vi "MB Serial Example Slave.vi"() -> ()   [LabVIEW 2019, in "NI_modbus_upd.lvlib"]
uses:
  NI_modbus_upd.lvlib
  MB Globals.vi
panel:
  in  "Stop":bool
  out "Holding Registers":u16[](array[numeric]) caption="Holding Registers (Master can write in these registers)"
  out "Coils":bool[](array[boolean]) caption="Coils (Master can write coils)"
  in  "Discrete Inputs":bool[](array[boolean]) caption="Discrete Inputs (Master can only read them)"
  in  "Input Registers":u16[](array[numeric]) caption="Input Registers (Master can only read them)"
  in  "VISA resource name":refnum<visa-resource-name>
  # "MB Serial Example Slave.vi\n\nInstructions\n1. Connect your 2 COMs ports using a cross-over cable\n2. Select a COM port in VISA resouce name\n3. Run the VI\n4. Open and run MB Example Master.vi\n5. Modify the discrete inputs or input registers on the slave -> they're updated on the master.\n6. Modify the coils and registers on the master -> they're updated on the slave."
  # "Slave Registers"
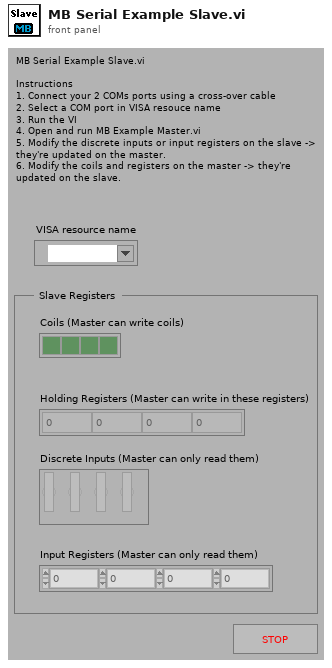
[diagram p1: front panel]
types:
  T1 = enum16{"Discrete Inputs", "Coils", "Input Registers", "Holding Registers"}
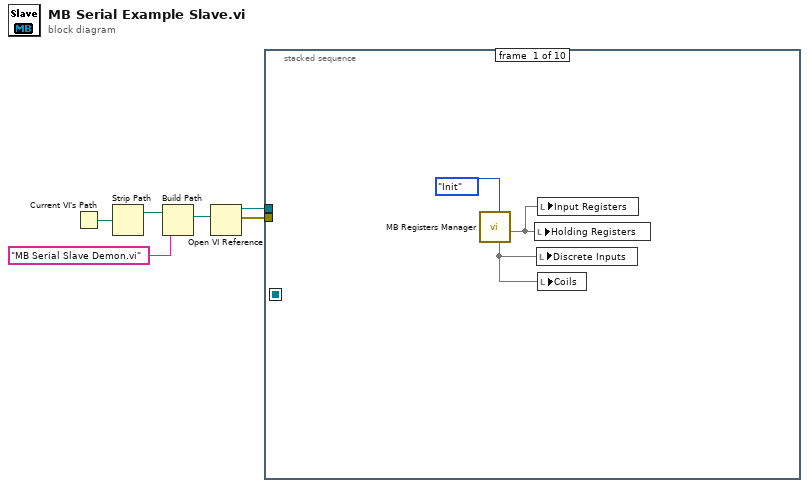
[diagram p0: block diagram]
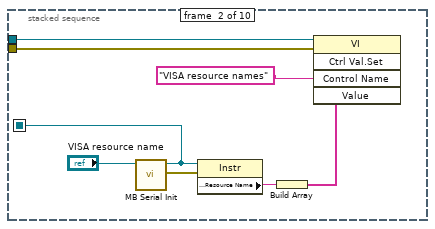
[diagram p2: hidden frame]
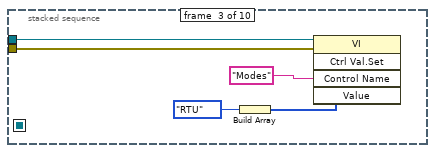
[diagram p3: hidden frame]
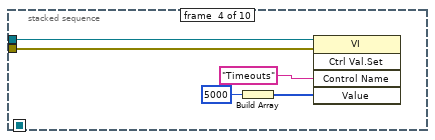
[diagram p4: hidden frame]
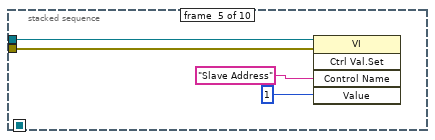
[diagram p5: hidden frame]
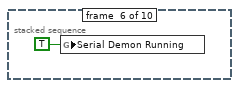
[diagram p6: hidden frame]
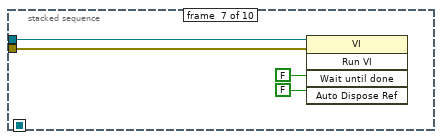
[diagram p7: hidden frame]
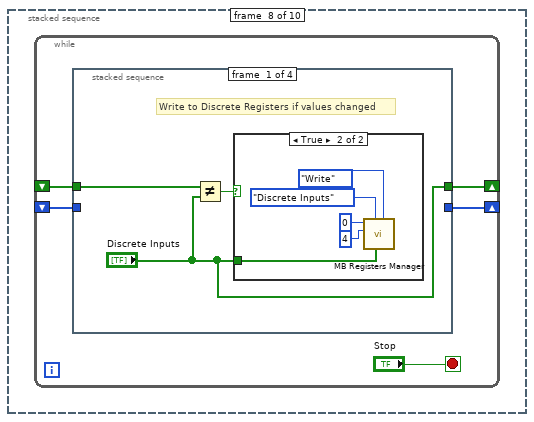
[diagram p8: hidden frame]
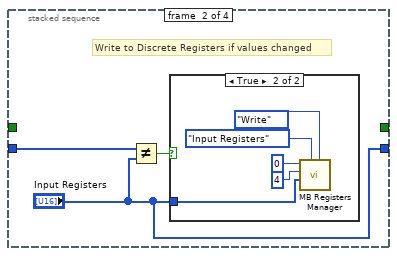
[diagram p10: hidden frame]
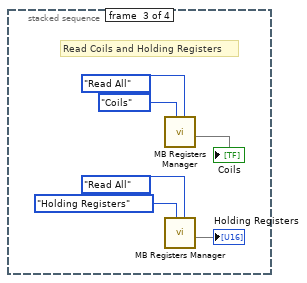
[diagram p12: hidden frame]
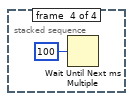
[diagram p13: hidden frame]
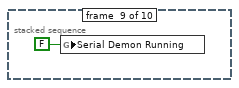
[diagram p14: hidden frame]
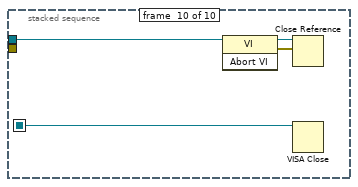
[diagram p15: hidden frame]
diagram:
  n1 = Current VI's Path() -> (path=w6:path)
  n2 = Strip Path(path=w6) -> (stripped path=w5:path)  [unwired: 1 out]
  n3 = Build Path(base path=w5, name or relative path="MB Serial Slave Demon.vi") -> (appended path=w3:path)
  n4 = Open VI Reference(vi path=w3) -> (vi reference=w2:refnum<vi>, error out=w1:errorcluster)  [unwired: 5 in]
  n5 = stacked-sequence {
    seq-local: [_ w13 _ _ _ _ _ _ _ _] -> [_ _ _ _ _ _ _ _ _ w69]
    tunnel: w2 -> [_ w16 w22 w27 w31 _ w36 _ _ w68]
    tunnel: w1 -> [_ w15 w21 w26 w30 _ w35 _ _ _]
    frame #0 {
      n6 = call "MB Registers Manager.vi"(5:enum16{"Init", "Read", "Write", "Read All"}."Init" ("Function")) -> (1:w8, 4:w7)  [unwired: 8 in, 1 out]
      n7 = local write "Holding Registers"(w8) -> ()
      n8 = local write "Discrete Inputs"(w7) -> ()
      n9 = local write "Input Registers"(w8) -> ()
      n10 = local write "Coils"(w7) -> ()
    }
    frame #1 {
      n11 = call "MB Serial Init.vi"("VISA resource name"="VISA resource name") -> ("error out"=w12:errorcluster, "VISA resource name out"=w13:refnum<visa-resource-name>)  [unwired: 9 in]
      n12 = property class="Instr"(reference=w13, error in=w12) -> ("General Settings:Resource Name"=w11:string)  [unwired: 2 out]
      n13 = Build Array(w11) -> (w10:string[])
      n14 = invoke class="VI" method="Ctrl Val.Set"(reference=w16, error in=w15, "Control Name"="VISA resource names", "Value"=w10) -> ()  [unwired: 1 in, 5 out]
    }
    frame #2 {
      n15 = Build Array(enum16{"RTU", "ASCII"}."RTU" ("Mode")) -> (w18:enum16{"RTU", "ASCII"}[])
      n16 = invoke class="VI" method="Ctrl Val.Set"(reference=w22, error in=w21, "Control Name"="Modes", "Value"=w18) -> ()  [unwired: 1 in, 5 out]
    }
    frame #3 {
      n17 = Build Array(u32 5000 ("Timeout")) -> (w23:u32[])
      n18 = invoke class="VI" method="Ctrl Val.Set"(reference=w27, error in=w26, "Control Name"="Timeouts", "Value"=w23) -> ()  [unwired: 1 in, 5 out]
    }
    frame #4 {
      n19 = invoke class="VI" method="Ctrl Val.Set"(reference=w31, error in=w30, "Control Name"="Slave Address", "Value"=u8 1 ("Slave Address")) -> ()  [unwired: 1 in, 5 out]
    }
    frame #5 {
      n20 = global write "MB Globals.vi" "Serial Demon Running"(TRUE ("Slave Demon Running")) -> ()
    }
    frame #6 {
      n21 = invoke class="VI" method="Run VI"(reference=w36, error in=w35, "Wait until done"=FALSE, "Auto Dispose Ref"=FALSE) -> ()  [unwired: 1 in, 5 out]
    }
    frame #7 {
      n22 = while {
        shift-right: [w40] -> _
        shift-left: _ -> [w39]
        shift-right: [w37] -> _
        shift-left: _ -> [w38]
        stop <- "Stop" stop-if-true
        n23 = stacked-sequence {
          tunnel: ["Discrete Inputs" _ _ _] -> w40
          tunnel: w39 -> [w44 _ _ _]
          tunnel: w38 -> [_ w51 _ _]
          tunnel: [_ "Input Registers" _ _] -> w37
          frame #0 {
            # "Write to Discrete Registers if values changed"
            n24 = Not Equal?(x=w44, y="Discrete Inputs") -> (x != y?=w42:bool)
            n25 = case shown="True" w42 {
              tunnel: "Discrete Inputs" -> [_ w45]
              frame False {
              }
              frame True {
                n26 = call "MB Registers Manager.vi"(5:enum16{"Init", "Read", "Write", "Read All"}."Write" ("Function"), "Bits In"=w45, "Table"=T1."Discrete Inputs", "Length"=u16 4, "Start Address"=u16 0) -> ()  [unwired: 6 in, 1 out]
              }
            }
          }
          frame #1 {
            # "Write to Discrete Registers if values changed"
            n27 = Not Equal?(x=w51, y="Input Registers") -> (x != y?=w52:bool)
            n28 = case shown="True" w52 {
              tunnel: "Input Registers" -> [_ w53]
              frame False {
              }
              frame True {
                n29 = call "MB Registers Manager.vi"(5:enum16{"Init", "Read", "Write", "Read All"}."Write" ("Function"), "Table"=T1."Input Registers", "Words In"=w53, "Length"=u16 4, "Start Address"=u16 0) -> ()  [unwired: 6 in, 1 out]
              }
            }
          }
          frame #2 {
            # "Read Coils and Holding Registers"
            n30 = call "MB Registers Manager.vi"(5:enum16{"Init", "Read", "Write", "Read All"}."Read All" ("Function"), "Table"=T1."Coils") -> (4:→"Coils")  [unwired: 8 in, 1 out]
            n31 = call "MB Registers Manager.vi"(5:enum16{"Init", "Read", "Write", "Read All"}."Read All" ("Function"), "Table"=T1."Holding Registers") -> (1:→"Holding Registers")  [unwired: 8 in, 1 out]
          }
          frame #3 {
            n32 = Wait Until Next ms Multiple(millisecond multiple=u32 100) -> ()  [unwired: 1 out]
          }
        }
      }
    }
    frame #8 {
      n33 = global write "MB Globals.vi" "Serial Demon Running"(FALSE ("Slave Demon Running")) -> ()
    }
    frame #9 {
      n34 = invoke class="VI" method="Abort VI"(reference=w68) -> (reference out=w67:refnum<vi>, error out=w66:errorcluster)  [unwired: 2 in, 1 out]
      n35 = Close Reference(reference=w67, error in (no error)=w66) -> ()  [unwired: 1 out]
      n36 = VISA Close(VISA resource name=w69) -> ()  [unwired: 1 in, 1 out]
    }
  }
